vi "Dashboard Main.vi"() -> ()   [LabVIEW 2014]
uses:
  <vilib>/event_ctls.llb/eventvkey.ctl
  <vilib>/Rock Robotics/WPI/Dashboard/WPI_DashboardLogging Global.vi
  <vilib>/Rock Robotics/Network Tables/SD Write Numeric Array.vi
  <vilib>/Rock Robotics/Network Tables/SD Read Number.vi
  <vilib>/Rock Robotics/Network Tables/SD Write Number.vi
  <vilib>/Utility/config.llb/Write Key (String).vi
  <vilib>/Utility/config.llb/Write Key (I32).vi
  <vilib>/Utility/config.llb/NI_LVConfig.lvlib
panel:
  out "RobotIP":string
  in  "TCP":refnum<k5>
  in  "Rec Mode":enum32{"Stop", "Record", "Playback"}(radio)
  in  "Vision":u16(ring)=3 items=["Camera Off", "USB Camera SW", "USB Camera HW", "IP Camera"]
  out "Camera IP":string
  out "Image Message":string="Timeout in Camera Communications"
  in  "Dashboard Tab":T1(tab)
  in  "Switch cameras":bool
  in  "Ring Light Color":T2={"Hue"={42.0, 143.0}, "Sat"={103.21428571428572, 255.0}, "Val"={103.0, 255.0}} {"Hue" scale=0.0..255.0 scale format="%#_3g"}
  in  "Switch to Binary":bool
  in  "Camera Settings":T3={"Frame Rate"=30, "Compression"=30, "Size"=1} {"Frame Rate" scale=1.0..30.0; "Size" items=["640x480", "320x240", "160x120"]}
  out "MotorChart R":cluster{"Numeric":dbl, "Numeric":dbl}(graph)
  out "MotorChart L":T4(graph)
  out "MotorSliders R":cluster{"MotorSlide1":dbl, "MotorSlide2":dbl} {"MotorSlide2" scale=-1.0..1.0 scale format="%#_2e"; "MotorSlide1" scale=-1.0..1.0 scale format="%#_2e"}
  out "MotorSliders L":T5 {"MotorSlide4 2" scale=0.0..14.0 scale format="%#_2e"; "MotorSlide2" scale=-1.0..1.0 scale format="%#_2e"; "MotorSlide1" scale=-1.0..1.0 scale format="%#_2e"}
  out "JS1 Z":dbl(slide) scale=-1.0..1.0 scale format="%#_2e"
  out "JS1 Graph":cluster{"X":dbl, "Y":dbl}[](graph)
  out "JS1 Buttons":T6
  out "JS2 Z":dbl(slide) scale=-1.0..1.0 scale format="%#_2e"
  out "JS2 Graph":cluster{"X":dbl, "Y":dbl}[](graph)
  out "JS2 Buttons":T6
  out "Mode":T7(ring)=enum."Auto Disabled"
  in  "DB Camera Config":bool
  out "fps":dbl format="%#.1g"
  out "Mbps":dbl format="%#.1g"
  out "Mbps 2":bool
  in  "DB/String 9":string
  in  "DB/String 8":string
  in  "DB/String 7":string
  in  "DB/String 6":string
  in  "DB/String 5":string
  in  "DB/String 4":string
  in  "DB/String 3":string
  in  "DB/String 2":string
  in  "DB/String 1":string
  in  "DB/String 0":string
  in  "DB/Slider 0":dbl(slide) scale=0.0..5.0
  in  "DB/Slider 1":dbl(slide) scale=0.0..5.0
  in  "DB/Slider 2":dbl(slide) scale=0.0..5.0
  in  "DB/Slider 3":dbl(slide) scale=0.0..5.0
  out "DB/LED 3":bool
  out "DB/LED 2":bool
  out "DB/LED 1":bool
  out "DB/LED 0":bool
  in  "DB/Button 3":bool
  in  "DB/Button 2":bool
  in  "DB/Button 1":bool
  in  "DB/Button 0":bool caption="New Name"
  out "gyro":dbl
  in  "# totes":dbl=1.0
  out "ultrasonic":dbl
  out "pot value":dbl
  in  "lift pid gains":dbl[](array[numeric])=[5.0, 0.0, 0.0]
  in  "Min lift output":dbl=0.2
  out "VROOM METER":dbl(knob) scale=0.0..10.0
  in  "Level setpoints":dbl[](array[numeric])=[0.6, 0.64, 0.79, 0.85]
  in  "lift lower limit":dbl=0.59
  in  "lift upper limit":dbl=0.86
  in  "proportional constant":dbl=11.0
  in  "Test Slider":dbl(slide) scale=0.0..100.0 scale format="%#_3g"
  in  "On/Off":bool caption="Solenoid"
  in  "Test Name":u16(ring) items=["Select the test to run...", "Example Test", "-------------------------------", "List of tests is built in robot code.", "Replace with your own automated tests."]
  in  "Test Tree":string(tree)
  in  "Motor":cluster{"Value":dbl, "Enable":bool} {"Value" scale=-1.0..1.0 scale format="%#_3g"}
  out "Progress":T8 {"Test Progress" scale=0.0..100.0}
  in  "Rev/Fwd":cluster{"Forward":bool, "Reverse":bool}
  in  "Test Ring":u16(ring) items=["Monochrome", "Color"]
  in  "Listbox":i32(listbox)
  out "Tree":string(tree)
  out "Camera Image":T9(plugin-control)
  out "Boolean":bool
  # "Left"
  # "Front"
  # "Right"
  # "Battery"
  # ":l"
  # ":)"
  # ":D"
  # ":/"
  # "VROOM!!!!!!"
  # ":("
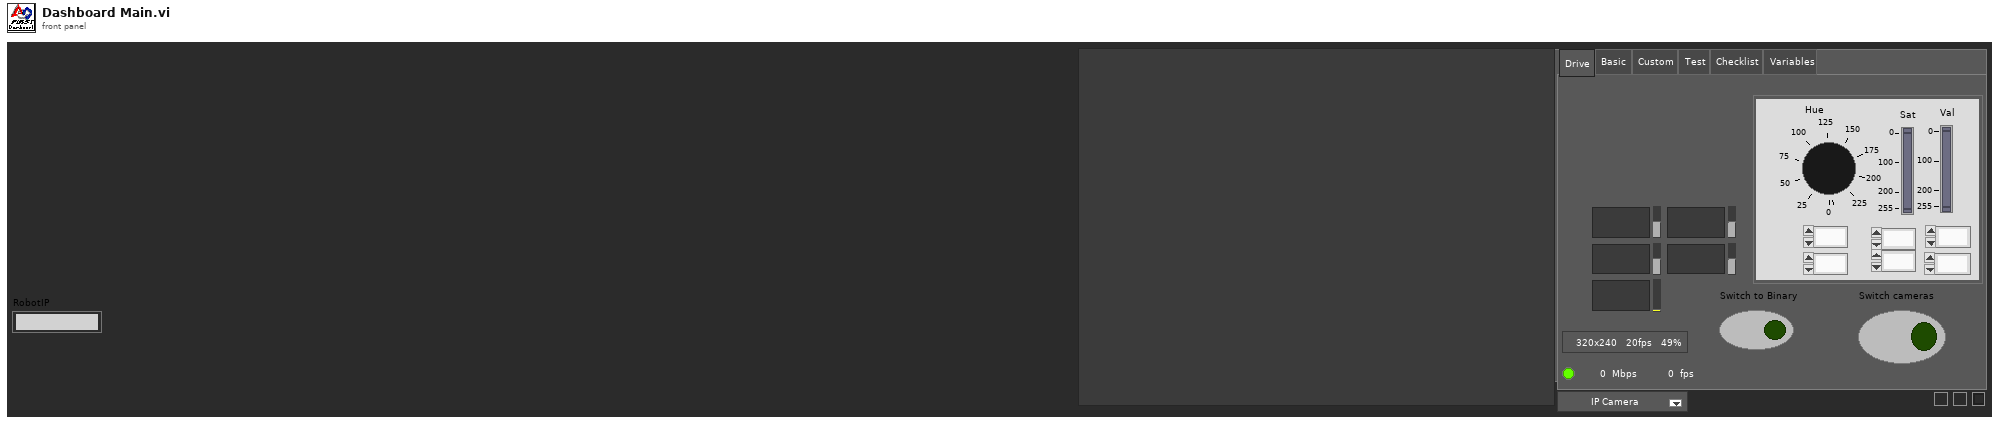
[diagram p1: front panel]
types:
  T1 = enum32{"Drive", "Basic", "Custom", "Test", "Checklist", "Variables"}
  T2 = cluster{"Hue":cluster{dbl, dbl}, "Sat":cluster{dbl, dbl}, "Val":cluster{dbl, dbl}}
  T3 = cluster{"Frame Rate":i32, "Compression":i32, "Size":u16}
  T4 = cluster{"Numeric":dbl, "Numeric":dbl, "Battery V":dbl}
  T5 = cluster{"MotorSlide1":dbl, "MotorSlide2":dbl, "MotorSlide4 2":dbl}
  T6 = cluster{bool, bool, bool, bool, bool, bool, bool, bool, bool, bool, bool, bool}
  T7 = enum8{"Tele-Op Disabled", "Tele-Op Enabled", "Auto Disabled", "Auto Enabled", "Test Disabled", "Test Enabled", "Disconnected", "No Code", "E-Stop"}
  T8 = cluster{"Test Progress":u8, "Test Progress Text":string}
  T9 = typedef "IMAQ Image.ctl" = refnum<image>
  T10 = typedef "Image Type" = u32
  T11 = cluster{"Camera Image":refnum<vi>, "Dashboard Tab":refnum<vi>, "Boolean":refnum<vi>, "Vision":refnum<vi>, "Rec Mode":refnum<vi>, "Test Slider":refnum<vi>, "On/Off ":refnum<vi>, "Test Ring":refnum<vi>, "Rev/Fwd":refnum<vi>, "Test Name":refnum<vi>, "Motor":refnum<vi>, "Progress":refnum<vi>, "CheckList":refnum<vi>, "Tree":refnum<vi>, "Test Tree":refnum<vi>}
  T12 = cluster{"Total Center of Mass":cluster{"X":dbl, "Y":dbl}, "average distance":dbl}
  T13 = cluster{"Error Strings":string, "Disable Counts":cluster{u16, u16}, "Rail Faults":cluster{u16, u16, u16}, "Robot IP":string, "DB Mode":u8, "Event Info":cluster{"Name":string, "Type":u8, "Number":u16, "Replay":u8}, "Camera Addr":string}
  T14 = cluster{"Storage":cluster{"Disk Free":u64, "RAM Block":u32, "RAM free":u32}, "CPU Utilization":cluster{"CPU % ISR":sgl, "CPU % Time Crit":sgl, "CPU % Timed Str":sgl, "CPU % High":sgl, "CPU % Above":sgl, "CPU % Normal":sgl, "CPU % Low":sgl}, "CAN":cluster{"% Bus Utilization":sgl, "Bus Off Cnt":u32, "TX_FIFO Full Cnt":u32, "Receive Error Cnt":u8, "Transmit Error Cnt":u8}, "HID":cluster{"HID Outputs":u32, "Rumble Low":u16, "Rumble High":u16}[]}
  T15 = cluster{"Status bits":cluster{"Test Mode":bool, "Autonomous":bool, "Enabled":bool, "Code Start":bool, "Brownout":bool, "Reserved 2":bool, "Reserved 3":bool, "E-Stop":bool}, "Code Trace":cluster{"Disabled":bool, "TeleOp":bool, "Auto":bool, "Test":bool}, "Controller Type":enum16{"unknown", "cRIO", "roboRio"}, "Code?":enum16{"unknown", "noCode", "code"}, "Battery V":dbl}
  T16 = cluster{"Control Bits":cluster{"TestMode":bool, "Autonomous":bool, "Enabled":bool, "FMS Present":bool, bool, bool, bool, "E-Stop":bool}, "Team Station ":u8, "Countdown":sgl, "Joystick Values":cluster{"Axes":dbl[], "Buttons":bool[], "POVs":i16[]}[]}
  T17 = cluster{"Axes":dbl[], "Buttons":bool[], "POVs":i16[]}[]
  T18 = cluster{"Axes":dbl[], "Buttons":bool[], "POVs":i16[]}
  T19 = cluster{"Buttons[0]":bool, "Buttons[1]":bool, "Buttons[2]":bool, "Buttons[3]":bool, "Buttons[4]":bool, "Buttons[5]":bool, "Buttons[6]":bool, "Buttons[7]":bool, "Buttons[8]":bool, "Buttons[9]":bool, "Buttons[10]":bool, "Buttons[11]":bool}
  T20 = typedef "NI_LVConfig.lvlib/Config Data RefNum.ctl" = refnum<k1>
  T21 = cluster{"Operation":enum16{"Update", "Clear"}, "Color Box":u32}[]
  T22 = typedef "eventvkey.ctl" = enum16{"ASCII", "Enter", "Return", "Shift", "Ctrl", "Alt", "Cmd", "Opt", "Caps", "NumLock", "Clear", "Break", "Up", "Down", "Left", "Right", "Insert", "Delete", "Home", "End", "PageUp", "PageDown", "Escape", "Help", "Pause", "ScrollLock", "F1", "F2", "F3", "F4", "F5", "F6", "F7", "F8", "F9", "F10", "F11", "F12", "F13", "F14", "F15", "F16", "F17", "F18", "F19", "F20", "F21", "F22", "F23", "F24", "Play", "VolumeUp", "VolumeDown", "Mute", "Two Byte Char"}
  T23 = cluster{"Image Size":bool, "Image Type":bool, "Pixel Value":bool, "ROI Information":bool, "Zoom Factor":bool}
  T24 = enum8{"Enabled", "Disabled", "Disabled and Grayed Out"}
  T25 = cluster{"Operation":enum16{"Update", "Clear"}, "Color Box":u32}
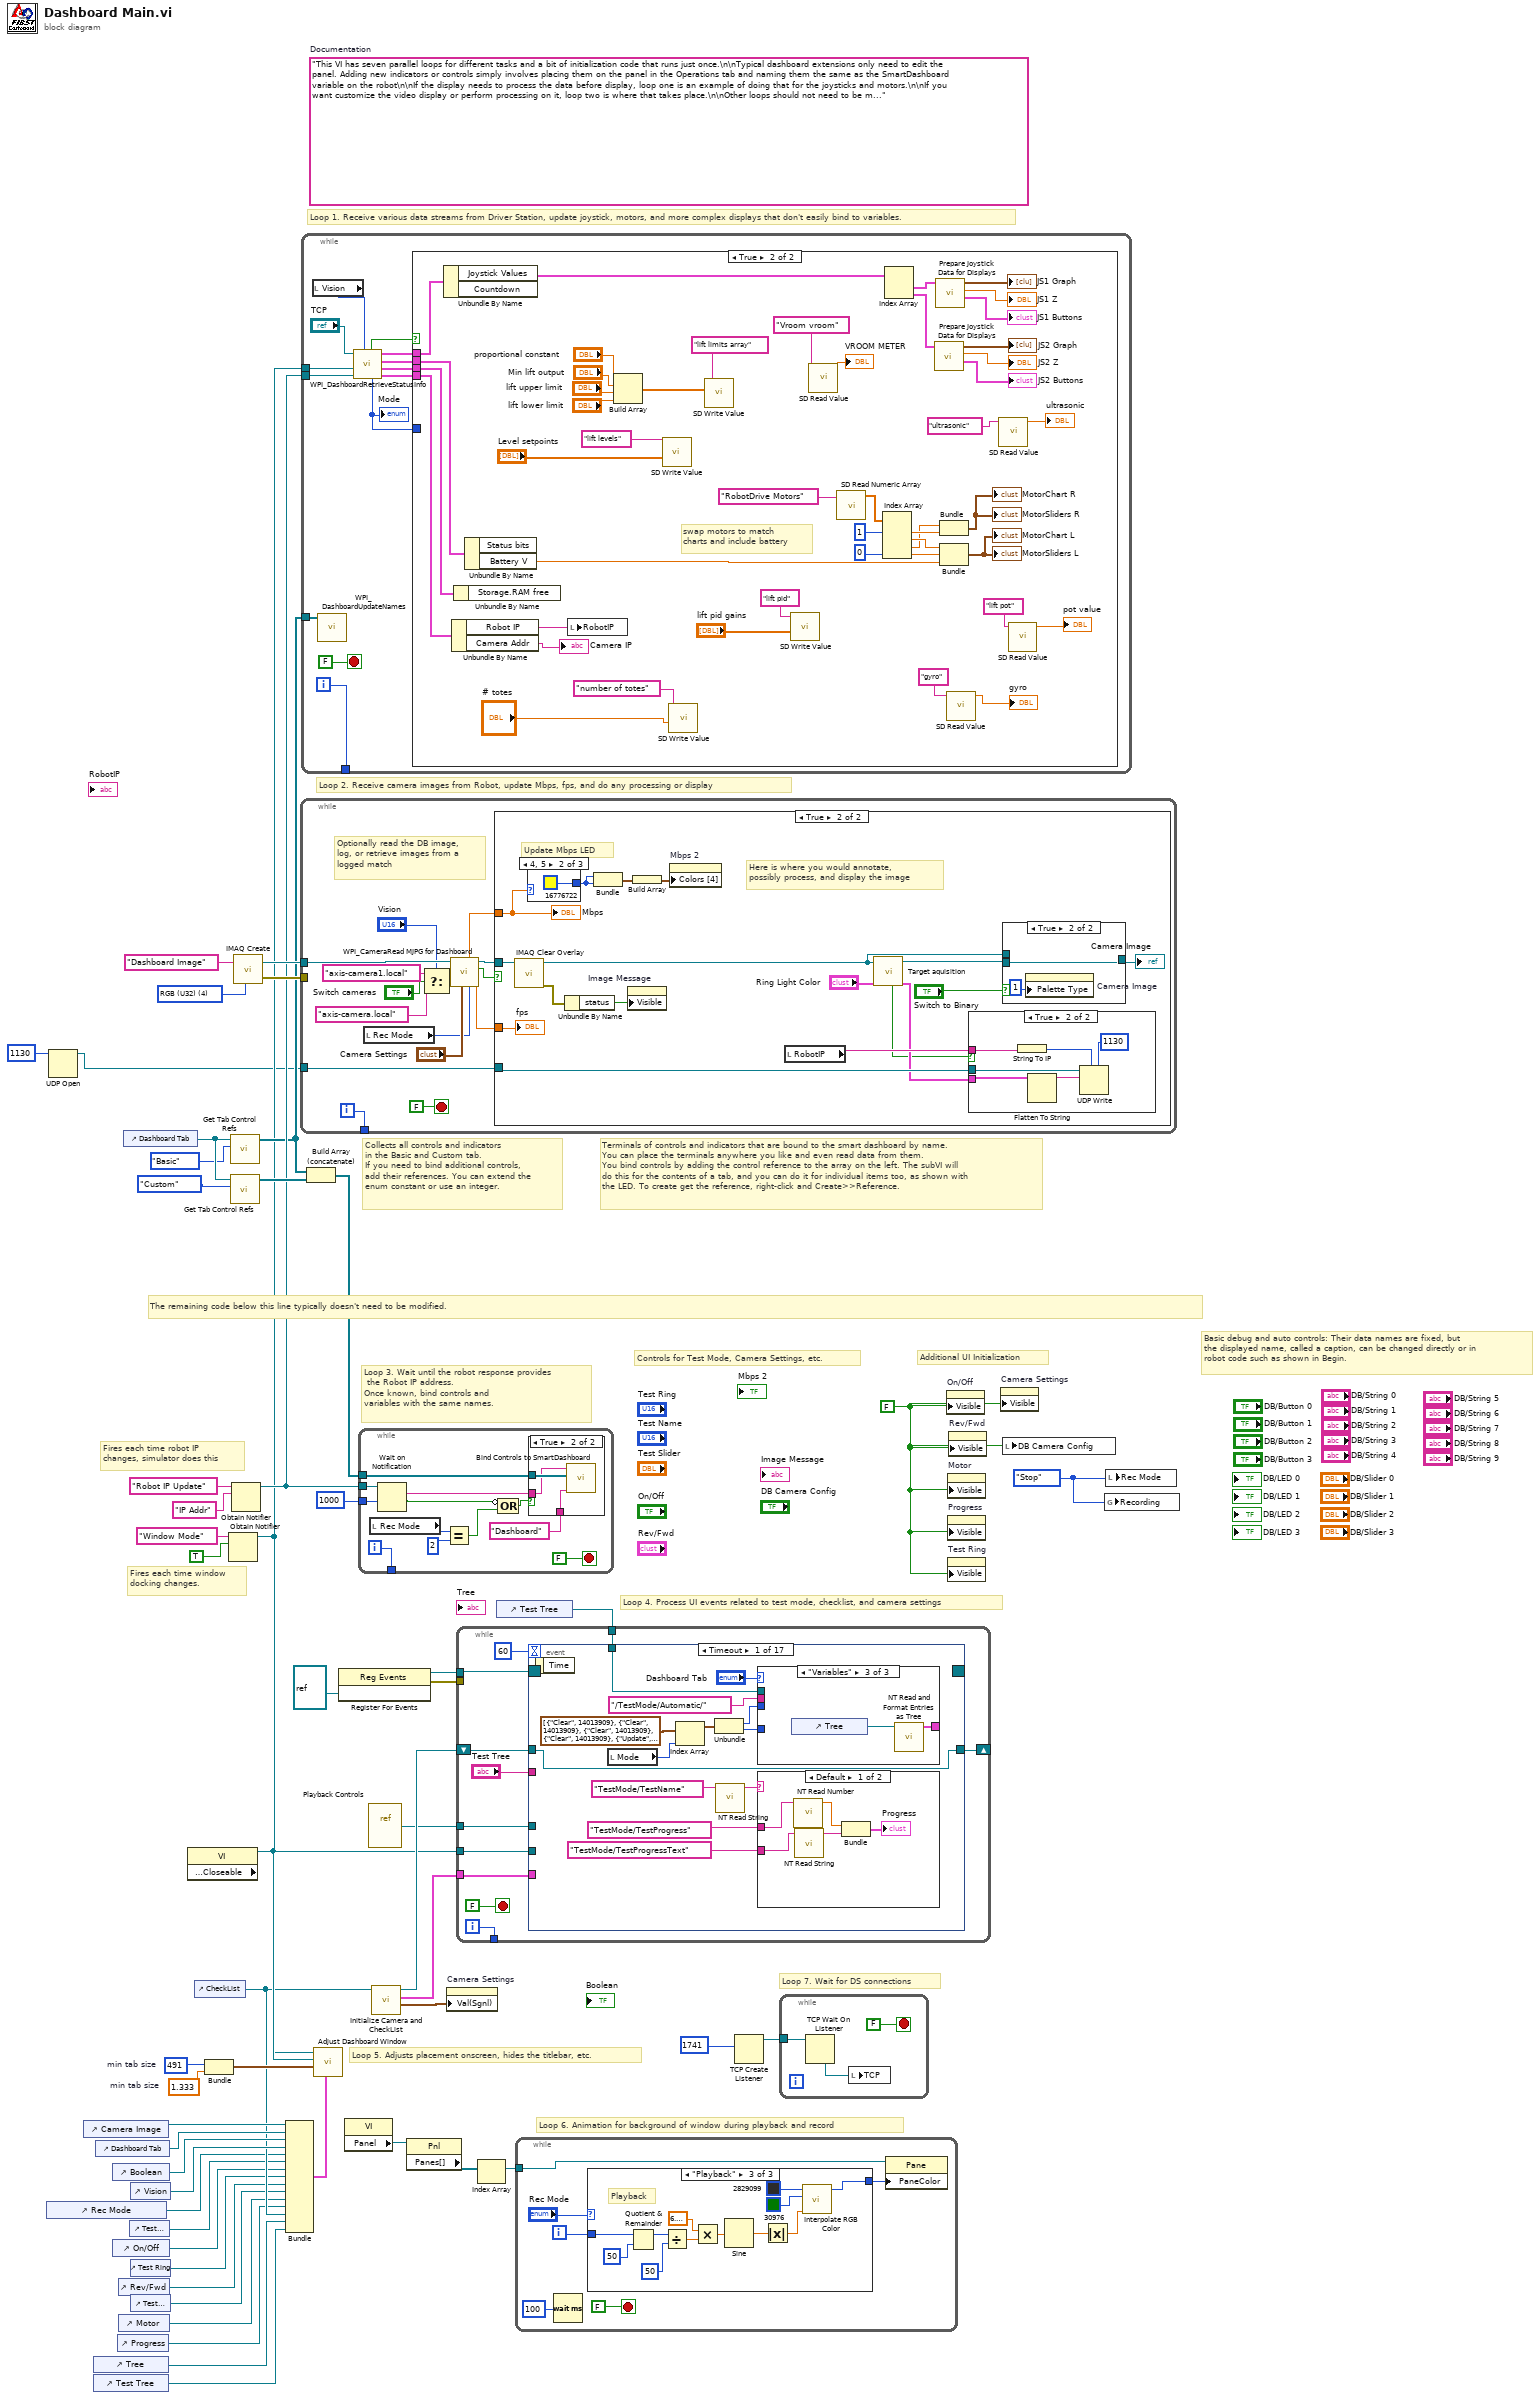
[diagram p0: block diagram]
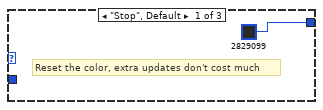
[diagram p3: hidden frame]
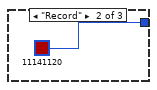
[diagram p4: hidden frame]
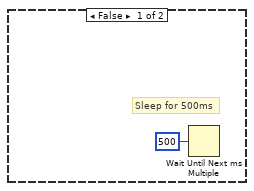
[diagram p6: hidden frame]
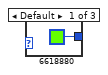
[diagram p9: hidden frame]
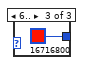
[diagram p10: hidden frame]
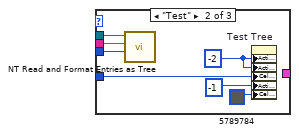
[diagram p12: hidden frame]
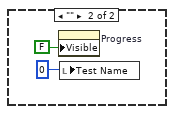
[diagram p13: hidden frame]
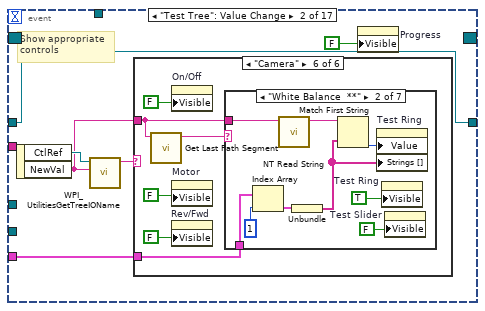
[diagram p14: hidden frame]
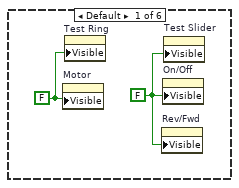
[diagram p15: hidden frame]
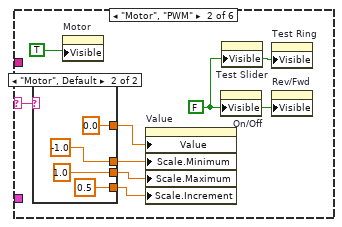
[diagram p16: hidden frame]
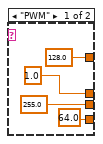
[diagram p17: hidden frame]
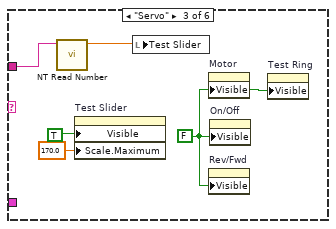
[diagram p18: hidden frame]
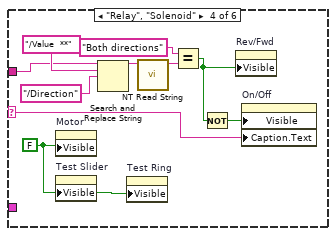
[diagram p19: hidden frame]
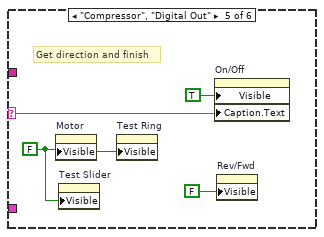
[diagram p20: hidden frame]
diagram:
  w26 = 491  # min tab size
  w25 = 1.333  # min tab size
  w34 = enum32{"Stop", "Record", "Playback"}."Stop" ("Rec Mode")
  w8 = FALSE ("Visible")
  (unwired) "This VI has seven parallel loops for different tasks and a bit of initialization code that runs just once.\n\nTypical dashboard extensions only need to edit the panel. Adding new indicators or controls simply involves placing them on the panel in the Operations tab and naming them the same as the SmartDashboard variable on the robot\n\nIf the display needs to process the data before display, loop one is an example of doing that for the joysticks and motors.\n\nIf you want customize the video display or perform processing on it, loop two is where that takes place.\n\nOther loops should not need to be modified. They are pretty standard, and document the task they perform."  # Documentation
  w54 = T10 4 items=["Grayscale (U8)", "Grayscale (I16)", "Grayscale (SGL)", "Complex (CSG)", "RGB (U32)", "HSL (U32)", "RGB (U64)"] ("Image Type")
  # "Loop 7. Wait for DS connections"
  # "Basic debug and auto controls: Their data names are fixed, but\nthe displayed name, called a caption, can be changed directly or in\nrobot code such as shown in Begin."
  # "Controls for Test Mode, Camera Settings, etc."
  # "Additional UI Initialization"
  # "Loop 6. Animation for background of window during playback and record"
  # "Fires each time robot IP\nchanges, simulator does this"
  # "Fires each time window\ndocking changes."
  # "Collects all controls and indicators\nin the Basic and Custom tab.\nIf you need to bind additional controls,\nadd their references. You can extend the\nenum constant or use an integer."
  # "The remaining code below this line typically doesn't need to be modified."
  # "Loop 4. Process UI events related to test mode, checklist, and camera settings"
  # "Terminals of controls and indicators that are bound to the smart dashboard by name.\nYou can place the terminals anywhere you like and even read data from them.\nYou bind controls by adding the control reference to the array on the left. The subVI will\ndo this for the contents of a tab, and you can do it for individual items too, as shown with\nthe LED. To create get the reference, right-click and Create>>Reference."
  # "Loop 3. Wait until the robot response provides\n the Robot IP address.\nOnce known, bind controls and\nvariables with the same names."
  # "Loop 5. Adjusts placement onscreen, hides the titlebar, etc."
  # "Loop 1. Receive various data streams from Driver Station, update joystick, motors, and more complex displays that don't easily bind to variables."
  # "Loop 2. Receive camera images from Robot, update Mbps, fps, and do any processing or display"
  n1 = control-ref of="Rec Mode"() -> (w14:refnum<vi>)
  n2 = UDP Open(11:1130) -> (port=w1:refnum<k16>)  [unwired: 4 in, 2 out]
  n3 = control-ref of="Camera Image"() -> (w29:refnum<vi>)
  n4 = control-ref of="Tree"() -> (w18:refnum<vi>)
  n5 = control-ref of="Test Tree"() -> (w17:refnum<vi>)
  n6 = control-ref of="Dashboard Tab"() -> (w28:refnum<vi>)
  n7 = control-ref of="Boolean"() -> (w23:refnum<vi>)
  n8 = control-ref of="On/Off"() -> (w12:refnum<vi>)
  n9 = control-ref of="Progress"() -> (w9:refnum<vi>)
  n10 = control-ref of="Rev/Fwd"() -> (w10:refnum<vi>)
  n11 = control-ref of="Motor"() -> (w15:refnum<vi>)
  n12 = control-ref of="Dashboard Tab"() -> (w32:refnum<vi>)
  n13 = control-ref of="Test Slider"() -> (w13:refnum<vi>)
  n14 = control-ref of="Vision"() -> (w27:refnum<vi>)
  n15 = control-ref of="Test Ring"() -> (w11:refnum<vi>)
  n16 = control-ref of="Test Name"() -> (w16:refnum<vi>)
  n17 = property class="VI" props=["Front Panel.Closeable"]() -> (reference out=w33:refnum<vi>)  [unwired: 2 in, 2 out]
  n18 = control-ref of="CheckList"() -> (w19:refnum<vi>)
  n19 = Bundle("min tab size"=w26, "min tab size"=w25) -> (w24:cluster{"min tab size":i32, "min tab size":dbl})  [unwired: 1 in]
  n20 = Obtain Notifier(name (unnamed)="Window Mode", notification data type=TRUE) -> (notifier out=w5:refnum<notifier>)  [unwired: 2 in, 2 out]
  n21 = call <vilib>:"Get Tab Control Refs.vi"("Page Index"=T1."Basic" ("Dashboard Tab"), "TabControl in"=w32) -> ("ControlsOnPage"=w6:refnum<vi>[])  [unwired: 9 in]
  n22 = call <vilib>:"Get Tab Control Refs.vi"("Page Index"=T1."Custom" ("Dashboard Tab"), "TabControl in"=w32) -> ("ControlsOnPage"=w31:refnum<vi>[])  [unwired: 9 in]
  n23 = Obtain Notifier(name (unnamed)="Robot IP Update", notification data type="IP Addr" ("name (unnamed)")) -> (notifier out=w7:refnum<notifier>)  [unwired: 2 in, 2 out]
  n24 = call "IMAQ Create"("Image Name"="Dashboard Image", "Image Type"=w54) -> ("New Image"=w52:T9, "error out"=w51:errorcluster)  [unwired: 2 in, 1 out]
  n25 = Bundle("Camera Image"=w29, "Dashboard Tab"=w28, "Boolean"=w23, "Vision"=w27, "Rec Mode"=w14, "Test Slider"=w13, "On/Off"=w12, "Test Ring"=w11, "Rev/Fwd"=w10, "Test Name"=w16, "Motor"=w15, "Progress"=w9, "CheckList"=w19, "Tree"=w18, "Test Tree"=w17) -> (w20:T11)  [unwired: 1 in]
  n26 = while {
    tunnel: w52 -> [w67]
    tunnel: w51 -> [_]
    tunnel: [w68] -> _
    tunnel: w1 -> [w59]
    i -> [w68]
    stop <- FALSE stop-if-true
    # "Optionally read the DB image,\nlog, or retrieve images from a\nlogged match"
    n27 = local read "Rec Mode"() -> (w61:enum32{"Stop", "Record", "Playback"})
    n28 = Select(t="axis-camera1.local", s="Switch cameras", f="axis-camera.local") -> (s? t:f=w58:string)
    n29 = call <vilib>:"WPI_CameraRead MJPG for Dashboard.vi"("Camera Settings"="Camera Settings", "Rec Mode"=w61, "Camera IP"=w58, "Camera Mode"="Vision", "Refnum in"=w67) -> ("Active"=w65:bool, "Refnum out"=w66:T9, "FPS"=w64:dbl, "Bandwidth (Mbps)"=w63:dbl)  [unwired: 3 in]
    n30 = case shown="True" w65 {
      tunnel: w66 -> [_ w82]
      tunnel: w63 -> [_ w81]
      tunnel: w64 -> [_ w80]
      tunnel: w59 -> [_ w73]
      frame False {
        # "Sleep for 500ms"
        n31 = Wait Until Next ms Multiple(millisecond multiple=u32 500) -> ()  [unwired: 1 out]
      }
      frame True {
        # "Here is where you would annotate,\npossibly process, and display the image"
        # "Update Mbps LED"
        n32 = call "IMAQ Clear Overlay"("Image"=w82) -> ("error out"=w86:errorcluster, "Image Out"=w78:T9)  [unwired: 2 in, 7 out]
        n33 = case shown="4, 5" w81 {
          tunnel: [u32 6618880 ("Color Box") u32 16776722 ("Color Box") u32 16716800 ("Color Box")] -> w83
          frame Default {
          }
          frame 4, 5 {
          }
          frame 6.. {
          }
        }
        n34 = Unbundle By Name(w86) -> ("status"=w87:bool)
        n35 = Bundle("Color Box"=w83, "Color Box"=w83) -> (w85:cluster{"Color Box":u32, "Color Box":u32})  [unwired: 1 out]
        n36 = property on="Image Message" class="Str"("Visible"=w87) -> ()  [unwired: 2 in, 2 out]
        n37 = Build Array(w85) -> (w84:cluster{"Color Box":u32, "Color Box":u32}[])
        n38 = property on="Mbps 2" class="Bool (strict)"("Colors [4]"=w84) -> ()  [unwired: 2 in, 2 out]
        n39 = local read "RobotIP"() -> (w74:string)
        n40 = call "Target aquisition.vi"("Ring Light Color"="Ring Light Color", "Image"=w78) -> ("Target tracking data"=w72:T12, "Threshold image"=w76:T9, "is there a target"=w71:bool)  [unwired: 7 in]
        n41 = case shown="True" w71 {
          tunnel: w74 -> [_ w91]
          tunnel: w73 -> [_ w90]
          tunnel: w72 -> [_ w88]
          frame False {
          }
          frame True {
            n42 = String To IP(1:w91) -> (0:w92:u32)
            n43 = Flatten To String(anything=w88) -> (data string=w93:string)  [unwired: 3 in, 2 out]
            n44 = UDP Write(address=w92, port or service name=1130, connection ID=w90, data in=w93) -> ()  [unwired: 2 in, 2 out]
          }
        }
        n45 = case shown="True" "Switch to Binary" {
          tunnel: w78 -> [w94 _]
          tunnel: [w94 w95] -> w77
          tunnel: w76 -> [_ w95]
          frame False {
          }
          frame True {
            n46 = property on="Camera Image" class="ImageControl"("Palette Type"=1) -> ()  [unwired: 2 in, 2 out]
          }
        }
        "Camera Image" <- w77
        "Mbps" <- w81
        "fps" <- w80
      }
    }
  }
  n47 = while {
    tunnel: [w111] -> _
    tunnel: w7 -> [w105]
    tunnel: w6 -> [w104]
    tunnel: w5 -> [w100]
    i -> [w111]
    stop <- FALSE stop-if-true
    n48 = local read "Vision"() -> (w102:u16)
    n49 = call <vilib>:"WPI_DashboardUpdateNames.vi"("Controls on Tab"=w104) -> ()  [unwired: 11 in]
    n50 = call <vilib>:"WPI_DashboardRetrieveStatusInfo.vi"("Vision"=w102, "Binding Refnum"=w105, "Window Mode Notifier"=w100, "TCP Cnx"="TCP") -> ("Power and Errors"=w106:T13, "Robot Metrics"=w109:T14, "Status Info"=w110:T15, "Control Info"=w107:T16, "Robot Mode"=w103:T7, "Process?"=w108:bool)  [unwired: 2 in]
    "Mode" <- w103
    n51 = case shown="True" w108 {
      tunnel: w110 -> [_ w158]
      tunnel: w109 -> [_ w157]
      tunnel: w107 -> [_ w156]
      tunnel: w106 -> [_ w155]
      tunnel: w103 -> [_ _]
      frame False {
      }
      frame True {
        # "swap motors to match\ncharts and include battery"
        n52 = Unbundle By Name(w156) -> ("Joystick Values"=w143:T17)  [unwired: 1 out]
        n53 = Unbundle By Name(w155) -> ("Robot IP"=w117:string, "Camera Addr"=→"Camera IP":string)
        n54 = Unbundle By Name(w157) -> ()  [unwired: 1 out]
        n55 = Unbundle By Name(w158) -> ("Battery V"=w144:dbl)  [unwired: 1 out]
        n56 = local write "RobotIP"(w117) -> ()
        n57 = Build Array("proportional constant", "Min lift output", "lift upper limit", "lift lower limit") -> (w130:dbl[])
        n58 = call-poly <vilib>:"SD Write Value.vi"("Numeric Array"="Level setpoints", "Name"="lift levels") -> ()  [unwired: 8 in, 2 out]
        n59 = call-poly <vilib>:"SD Write Value.vi"("Numeric"="# totes", "Name"="number of totes") -> ()  [unwired: 8 in, 2 out]
        n60 = call-poly <vilib>:"SD Write Value.vi"("Numeric Array"=w130, "Name"="lift limits array") -> ()  [unwired: 8 in, 2 out]
        n61 = call-poly <vilib>:"SD Write Value.vi"("Numeric Array"="lift pid gains", "Name"="lift pid") -> ()  [unwired: 8 in, 2 out]
        n62 = call-poly <vilib>:"SD Read Value.vi"("Name"="Vroom vroom") -> ("Numeric"=→"VROOM METER":dbl)  [unwired: 8 in, 2 out]
        n63 = call <vilib>:"SD Read Numeric Array.vi"("Name"="RobotDrive Motors") -> ("Numeric Array"=w146:dbl[])  [unwired: 8 in, 2 out]
        n64 = Index Array(array=w146, index #1=1, index #4=0) -> (element #1=w150:dbl, element #2=w151:dbl, element #3=w149:dbl, element #4=w154:dbl)  [unwired: 2 in]
        n65 = Index Array(array=w143) -> (element #1=w142:T18, element #2=w137:T18)  [unwired: 2 in]
        n66 = call "Prepare Joystick Data for Displays.vi"("Joystick Values"=w137) -> ("Buttons"=→"JS2 Buttons":T19, "Z Axis"=→"JS2 Z":dbl, "Cartesian Data"=→"JS2 Graph":cluster{"X axis":dbl, "X axis":dbl}[])  [unwired: 8 in]
        n67 = call "Prepare Joystick Data for Displays.vi"("Joystick Values"=w142) -> ("Buttons"=→"JS1 Buttons":T19, "Z Axis"=→"JS1 Z":dbl, "Cartesian Data"=→"JS1 Graph":cluster{"X axis":dbl, "X axis":dbl}[])  [unwired: 8 in]
        n68 = Bundle("Numeric"=w149, "Numeric"=w150) -> (→"MotorChart R" →"MotorSliders R":cluster{"Numeric":dbl, "Numeric":dbl})  [unwired: 1 in]
        n69 = Bundle("Numeric"=w151, "Numeric"=w154, "Battery V"=w144) -> (→"MotorChart L" →"MotorSliders L":T4)  [unwired: 1 in]
        n70 = call-poly <vilib>:"SD Read Value.vi"("Name"="gyro") -> ("Numeric"=→"gyro":dbl)  [unwired: 8 in, 2 out]
        n71 = call-poly <vilib>:"SD Read Value.vi"("Name"="ultrasonic") -> ("Numeric"=→"ultrasonic":dbl)  [unwired: 8 in, 2 out]
        n72 = call-poly <vilib>:"SD Read Value.vi"("Name"="lift pot") -> ("Numeric"=→"pot value":dbl)  [unwired: 8 in, 2 out]
      }
    }
  }
  n73 = Build Array (concatenate)(w6, w31) -> (w30:refnum<vi>[])
  n74 = call "Adjust Dashboard Window.vi"("Sizing Refnums"=w20, "Size Constraints"=w24, "VI"=w33, "Notifier in"=w5) -> ()  [unwired: 8 in]
  n75 = register-events(refnum<vi> refnum) -> (reference out=w38:refnum<event-registration>, error out=w37:errorcluster)  [unwired: 2 in]
  n76 = property class="VI"() -> ("Panel"=w41:refnum<vi>)  [unwired: 2 in, 2 out]
  n77 = while {
    tunnel: w30 -> [w170]
    tunnel: w7 -> [w168]
    tunnel: [w166] -> _
    tunnel: u32 1000 ("milliseconds to wait") -> [w165]
    i -> [w166]
    stop <- FALSE stop-if-true
    n78 = local read "Rec Mode"() -> (w161:enum32{"Stop", "Record", "Playback"})
    n79 = Wait on Notification(notifier=w168, timeout in ms (-1)=w165) -> (notification=w167:string, timed out?=w163:bool)  [unwired: 2 in, 2 out]
    n80 = Equal?(x=w161, y=u16 2 ("Rec Mode")) -> (x = y?=w162:bool)
    n81 = Compound Arithmetic op=OR(invert w163, w162) -> (w164:bool)
    n82 = case shown="True" w164 {
      tunnel: w170 -> [_ w173]
      tunnel: w167 -> [_ w172]
      tunnel: "Dashboard" -> [_ w171]
      frame False {
      }
      frame True {
        n83 = call <vilib>:"Bind Controls to SmartDashboard.vi"("Client Name"=w171, "Bound Control Refs"=w173, "Server IP Address"=w172) -> ()  [unwired: 9 in]
      }
    }
  }
  n84 = vi-ref "Playback Controls.vi"() -> (w39:refnum<vi>)
  n85 = call "Initialize Camera and CheckList.vi"("ListBox in"=w19) -> ("Cluster"=w45:cluster{"value":i32, "value":i32, "index":i32}, "Array"=w46:cluster{string[]}[], "File Refnum"=w44:T20)  [unwired: 8 in]
  n86 = property class="Pnl"(reference=w41) -> ("Panes[]"=w42:refnum<vi>[])  [unwired: 1 in, 2 out]
  n87 = property on="Camera Settings" class="Clust (strict)"("Val(Sgnl)"=w45) -> ()  [unwired: 2 in, 2 out]
  n88 = Index Array(array=w42) -> (element=w40:refnum<vi>)  [unwired: 1 in]
  n89 = control-ref of="Test Tree"() -> (w43:refnum<vi>)
  n90 = while {
    tunnel: w46 -> [w181]
    shift-right: [w180] -> _
    shift-left: w44 -> [w179]
    tunnel: [w178] -> _
    tunnel: w43 -> [w177]
    tunnel: w39 -> [w176]
    tunnel: w38 -> [w175]
    tunnel: w37 -> [_]
    tunnel: w33 -> [w174]
    i -> [w178]
    stop <- FALSE stop-if-true
    n91 = event shown="[0] Timeout" {
      selector: w175 -> [_ _ _ _ _ _ _ _ _ _ _ _ _ _ _ _ _]
      dyn-events: [_ _ _ _ _ _ _ _ _ _ _ _ _ w419 _ _ _] -> _
      timeout: u32 60 ("milliseconds to wait") -> [_ _ _ _ _ _ _ _ _ _ _ _ _ _ _ _ _]
      tunnel: w177 -> [w193 _ _ _ _ _ _ _ _ _ _ _ _ _ _ _ _]
      tunnel: "Test Tree" -> [_ _ _ _ _ _ _ _ w388 w396 w398 w402 w410 _ _ _ _]
      tunnel: w181 -> [_ w215 _ _ _ _ w352 w382 _ _ _ _ _ _ _ _ _]
      tunnel: [w189 w214 w313 w318 w326 w338 w351 w375 w387 w394 w397 w401 w409 w421 w435 w436 w446] -> w180
      tunnel: w179 -> [w189 w214 w313 w318 w326 w338 w350 w375 w387 w394 w397 w401 w409 w421 w435 w436 w446]
      tunnel: w176 -> [_ _ _ _ _ _ _ _ _ _ _ _ _ w422 _ w439 _]
      tunnel: w174 -> [_ _ _ _ _ _ _ _ _ _ _ _ _ w417 _ _ _]
      event Timeout {
        n92 = event-data() -> ()  [unwired: 1 in, 1 out]
        n93 = local read "Mode"() -> (w192:T7)
        n94 = Index Array(array=T21 [{"Operation"=enum."Clear", "Color Box"=14013909}, {"Operation"=enum."Clear", "Color Box"=14013909}, {"Operation"=enum."Clear", "Color Box"=14013909}, {"Operation"=enum."Clear", "Color Box"=14013909}, {"Operation"=enum."Update", "Color Box"=14013909}, {"Operation"=enum."Update", "Color Box"=16777215}, {"Operation"=enum."Clear", "Color Box"=14013909}, {"Operation"=enum."Clear", "Color Box"=14013909}, {"Operation"=enum."Clear", "Color Box"=14013909}], index=w192) -> (element=w187:T25)
        n95 = Unbundle(w187) -> ("Operation"=w186:enum16{"Update", "Clear"}, "Color Box"=w185:u32)
        n96 = call <vilib>:"NT Read String.vi"("Name"="TestMode/TestName") -> ("String"=w196:string)  [unwired: 9 in, 1 out]
        n97 = case shown="\"Variables\"" "Dashboard Tab" {
          tunnel: w193 -> [_ w204 _]
          tunnel: "/TestMode/Automatic/" ("Name Pattern") -> [_ w203 _]
          tunnel: w186 -> [_ w202 _]
          tunnel: [_ _ w206] -> _
          tunnel: w185 -> [_ w198 _]
          frame "Custom", Default {
          }
          frame "Test" {
            w201 = -2 ("Active Item:Row Number")
            n98 = call <vilib>:"NT Read and Format Entries as Tree.vi"("Operation"=w202, "Name Pattern"=w203, "Tree Refnum"=w204) -> ()  [unwired: 7 in, 2 out]
            n99 = property on="Test Tree" class="Tree (strict)"("Active Item Row Number"=w201, "ActiveColNum"=w201, "CellBG"=w198, "Active Item Row Number"=-1 ("Active Item:Row Number"), "CellBG"=u32 5789784 ("Color Box")) -> ()  [unwired: 2 in, 2 out]
          }
          frame "Variables" {
            n100 = control-ref of="Tree"() -> (w205:refnum<vi>)
            n101 = call <vilib>:"NT Read and Format Entries as Tree.vi"("Tree Refnum"=w205) -> ("Formatted Strings"=w206:cluster{"Name":string, "Value":string}[])  [unwired: 9 in, 1 out]
          }
        }
        n102 = case shown="Default" w196 {
          tunnel: "TestMode/TestProgress" ("Name") -> [w208 _]
          tunnel: "TestMode/TestProgressText" ("Name") -> [w207 _]
          frame Default {
            n103 = call <vilib>:"NT Read Number.vi"("Name"=w208) -> ("Numeric"=w209:dbl)  [unwired: 9 in, 1 out]
            n104 = call <vilib>:"NT Read String.vi"("Name"=w207) -> ("String"=w210:string)  [unwired: 9 in, 1 out]
            n105 = Bundle("Numeric"=w209, "String"=w210) -> (→"Progress":cluster{"Numeric":dbl, "String":string})  [unwired: 1 in]
          }
          frame "" {
            n106 = property on="Progress" class="Clust (strict)"("Visible"=FALSE) -> ()  [unwired: 2 in, 2 out]
            n107 = local write "Test Name"(u16 0) -> ()
          }
        }
      }
      event "Test Tree": Value Change {
        # "Show appropriate\ncontrols"
        n108 = event-data() -> ("CtlRef"=w218:refnum<vi>, "NewVal"=w216:string)  [unwired: 1 in]
        n109 = call <vilib>:"WPI_UtilitiesGetTreeIOName.vi"("NewVal"=w216, "TreeControl in"=w218) -> ("I/O Name"=w219:string)  [unwired: 9 in]
        n110 = case shown="\"Camera\"" w219 {
          selector: w219 -> [_ w226 _ w244 w253 _]
          tunnel: w216 -> [_ _ w241 w243 _ w260]
          tunnel: w215 -> [_ _ _ _ _ w259]
          frame Default {
            w221 = FALSE ("Visible")
            w220 = FALSE ("Visible")
            n111 = property on="Motor" class="Clust (strict)"("Visible"=w220) -> ()  [unwired: 2 in, 2 out]
            n112 = property on="Test Ring" class="Ring (strict)"("Visible"=w220) -> ()  [unwired: 2 in, 2 out]
            n113 = property on="Rev/Fwd" class="Clust (strict)"("Visible"=w221) -> ()  [unwired: 2 in, 2 out]
            n114 = property on="On/Off" class="Bool (strict)"("Visible"=w221) -> ()  [unwired: 2 in, 2 out]
            n115 = property on="Test Slider" class="Slide (strict)"("Visible"=w221) -> ()  [unwired: 2 in, 2 out]
          }
          frame "Motor", "PWM" {
            w227 = FALSE ("Visible")
            n116 = case shown="\"Motor\", Default" w226 {
              tunnel: [1.0 ("Value") -1.0 ("Value")] -> w225
              tunnel: [255.0 ("Value") 1.0 ("Value")] -> w224
              tunnel: [128.0 ("Value") 0.0 ("Value")] -> w223
              tunnel: [64.0 ("Value") 0.5 ("Value")] -> w222
              frame "PWM" {
              }
              frame "Motor", Default {
              }
            }
            n117 = property on="Motor" class="Clust (strict)"("Visible"=TRUE) -> ()  [unwired: 2 in, 2 out]
            n118 = property on="Value" class="Slide (strict)"("Value"=w223, "Scale.Minimum"=w225, "Scale.Maximum"=w224, "Scale.Increment"=w222) -> ()  [unwired: 2 in, 2 out]
            n119 = property on="On/Off" class="Bool (strict)"("Visible"=w227) -> ()  [unwired: 2 in, 2 out]
            n120 = property on="Test Slider" class="Slide (strict)"("Visible"=w227) -> ()  [unwired: 2 in, 2 out]
            n121 = property on="Test Ring" class="Ring (strict)"("Visible"=w227) -> ()  [unwired: 2 in, 2 out]
            n122 = property on="Rev/Fwd" class="Clust (strict)"("Visible"=w227) -> ()  [unwired: 2 in, 2 out]
          }
          frame "Servo" {
            w239 = FALSE ("Visible")
            n123 = call <vilib>:"NT Read Number.vi"("Name"=w241) -> ("Numeric"=w240:dbl)  [unwired: 9 in, 1 out]
            n124 = property on="Test Slider" class="Slide (strict)"("Visible"=TRUE, "Scale.Maximum"=170.0 ("Scale.Range:Maximum")) -> ()  [unwired: 2 in, 2 out]
            n125 = local write "Test Slider"(w240) -> ()
            n126 = property on="Motor" class="Clust (strict)"("Visible"=w239) -> ()  [unwired: 2 in, 2 out]
            n127 = property on="Rev/Fwd" class="Clust (strict)"("Visible"=w239) -> ()  [unwired: 2 in, 2 out]
            n128 = property on="On/Off" class="Bool (strict)"("Visible"=w239) -> ()  [unwired: 2 in, 2 out]
            n129 = property on="Test Ring" class="Ring (strict)"("Visible"=w239) -> ()  [unwired: 2 in, 2 out]
          }
          frame "Relay", "Solenoid" {
            w242 = FALSE ("Visible")
            n130 = property on="Motor" class="Clust (strict)"("Visible"=w242) -> ()  [unwired: 2 in, 2 out]
            n131 = property on="Test Slider" class="Slide (strict)"("Visible"=w242) -> ()  [unwired: 2 in, 2 out]
            n132 = Search and Replace String(input string=w243, search string="/Value  **", replace string="/Direction") -> (result string=w249:string)  [unwired: 5 in, 3 out]
            n133 = property on="Test Ring" class="Ring (strict)"("Visible"=w242) -> ()  [unwired: 2 in, 2 out]
            n134 = call <vilib>:"NT Read String.vi"("Name"=w249) -> ("String"=w247:string)  [unwired: 9 in, 1 out]
            n135 = Equal?(x="Both directions", y=w247) -> (x = y?=w245:bool)
            n136 = Not(x=w245) -> (.not. x?=w246:bool)
            n137 = property on="Rev/Fwd" class="Clust (strict)"("Visible"=w245) -> ()  [unwired: 2 in, 2 out]
            n138 = property on="On/Off" class="Bool (strict)"("Visible"=w246, "Caption.Text"=w244) -> ()  [unwired: 2 in, 2 out]
          }
          frame "Compressor", "Digital Out" {
            w252 = FALSE ("Visible")
            # "Get direction and finish"
            n139 = property on="Motor" class="Clust (strict)"("Visible"=w252) -> ()  [unwired: 2 in, 2 out]
            n140 = property on="Test Slider" class="Slide (strict)"("Visible"=w252) -> ()  [unwired: 2 in, 2 out]
            n141 = property on="Test Ring" class="Ring (strict)"("Visible"=w252) -> ()  [unwired: 2 in, 2 out]
            n142 = property on="On/Off" class="Bool (strict)"("Visible"=TRUE, "Caption.Text"=w253) -> ()  [unwired: 2 in, 2 out]
            n143 = property on="Rev/Fwd" class="Clust (strict)"("Visible"=FALSE) -> ()  [unwired: 2 in, 2 out]
          }
          frame "Camera" {
            n144 = call <vilib>:"Get Last Path Segment.vi"("String in"=w260) -> ("String out"=w261:string)  [unwired: 10 in]
            n145 = property on="On/Off" class="Bool (strict)"("Visible"=FALSE) -> ()  [unwired: 2 in, 2 out]
            n146 = property on="Motor" class="Clust (strict)"("Visible"=FALSE) -> ()  [unwired: 2 in, 2 out]
            n147 = property on="Rev/Fwd" class="Clust (strict)"("Visible"=FALSE) -> ()  [unwired: 2 in, 2 out]
            n148 = case shown="\"White Balance  **\"" w261 {
              tunnel: w260 -> [w267 w276 w285 w294 w303 _ w309]
              tunnel: w259 -> [w265 w273 w282 w291 w300 _ _]
              frame "Size  **" {
                n149 = Index Array(array=w265) -> (element=w264:cluster{string[]})  [unwired: 1 in]
                n150 = call <vilib>:"NT Read String.vi"("Name"=w267) -> ("String"=w266:string)  [unwired: 9 in, 1 out]
                n151 = Unbundle(w264) -> (w262:string[])
                n152 = Match First String(2:w262, 3:w266) -> (0:w263:i32)  [unwired: 1 out]
                n153 = property on="Test Ring" class="Ring (strict)"("Value"=w263, "Strings []"=w262) -> ()  [unwired: 2 in, 2 out]
                n154 = property on="Test Ring" class="Ring (strict)"("Visible"=TRUE) -> ()  [unwired: 2 in, 2 out]
                n155 = property on="Test Slider" class="Slide (strict)"("Visible"=FALSE) -> ()  [unwired: 2 in, 2 out]
              }
              frame "White Balance  **" {
                n156 = Index Array(array=w273, index=1) -> (element=w274:cluster{string[]})
                n157 = call <vilib>:"NT Read String.vi"("Name"=w276) -> ("String"=w275:string)  [unwired: 9 in, 1 out]
                n158 = Unbundle(w274) -> (w271:string[])
                n159 = Match First String(2:w271, 3:w275) -> (0:w270:i32)  [unwired: 1 out]
                n160 = property on="Test Ring" class="Ring (strict)"("Value"=w270, "Strings []"=w271) -> ()  [unwired: 2 in, 2 out]
                n161 = property on="Test Ring" class="Ring (strict)"("Visible"=TRUE) -> ()  [unwired: 2 in, 2 out]
                n162 = property on="Test Slider" class="Slide (strict)"("Visible"=FALSE) -> ()  [unwired: 2 in, 2 out]
              }
              frame "Exposure  **" {
                n163 = Index Array(array=w282, index=2) -> (element=w283:cluster{string[]})
                n164 = call <vilib>:"NT Read String.vi"("Name"=w285) -> ("String"=w284:string)  [unwired: 9 in, 1 out]
                n165 = Unbundle(w283) -> (w279:string[])
                n166 = Match First String(2:w279, 3:w284) -> (0:w280:i32)  [unwired: 1 out]
                n167 = property on="Test Ring" class="Ring (strict)"("Value"=w280, "Strings []"=w279) -> ()  [unwired: 2 in, 2 out]
                n168 = property on="Test Ring" class="Ring (strict)"("Visible"=TRUE) -> ()  [unwired: 2 in, 2 out]
                n169 = property on="Test Slider" class="Slide (strict)"("Visible"=FALSE) -> ()  [unwired: 2 in, 2 out]
              }
              frame "Exposure Priority  **" {
                n170 = Index Array(array=w291, index=3) -> (element=w292:cluster{string[]})
                n171 = call <vilib>:"NT Read String.vi"("Name"=w294) -> ("String"=w293:string)  [unwired: 9 in, 1 out]
                n172 = Unbundle(w292) -> (w288:string[])
                n173 = Match First String(2:w288, 3:w293) -> (0:w289:i32)  [unwired: 1 out]
                n174 = property on="Test Ring" class="Ring (strict)"("Value"=w289, "Strings []"=w288) -> ()  [unwired: 2 in, 2 out]
                n175 = property on="Test Ring" class="Ring (strict)"("Visible"=TRUE) -> ()  [unwired: 2 in, 2 out]
                n176 = property on="Test Slider" class="Slide (strict)"("Visible"=FALSE) -> ()  [unwired: 2 in, 2 out]
              }
              frame "Color Enable  **" {
                n177 = Index Array(array=w300, index=4) -> (element=w301:cluster{string[]})
                n178 = call <vilib>:"NT Read String.vi"("Name"=w303) -> ("String"=w302:string)  [unwired: 9 in, 1 out]
                n179 = Unbundle(w301) -> (w297:string[])
                n180 = Match First String(2:w297, 3:w302) -> (0:w298:i32)  [unwired: 1 out]
                n181 = property on="Test Ring" class="Ring (strict)"("Value"=w298, "Strings []"=w297) -> ()  [unwired: 2 in, 2 out]
                n182 = property on="Test Ring" class="Ring (strict)"("Visible"=TRUE) -> ()  [unwired: 2 in, 2 out]
                n183 = property on="Test Slider" class="Slide (strict)"("Visible"=FALSE) -> ()  [unwired: 2 in, 2 out]
              }
              frame Default {
                n184 = property on="Test Ring" class="Ring (strict)"("Visible"=FALSE) -> ()  [unwired: 2 in, 2 out]
                n185 = property on="Test Slider" class="Slide (strict)"("Visible"=FALSE) -> ()  [unwired: 2 in, 2 out]
              }
              frame "Brightness  **", "Color Level  **", "Compression  **", "FPS  **", "Sharpness  **" {
                n186 = call <vilib>:"NT Read Number.vi"("Name"=w309) -> ("Numeric"=w308:dbl)  [unwired: 9 in, 1 out]
                n187 = local write "Test Slider"(w308) -> ()
                n188 = property on="Test Slider" class="Slide (strict)"("Visible"=TRUE, "Scale.Maximum"=100.0 ("Scale.Range:Maximum")) -> ()  [unwired: 2 in, 2 out]
                n189 = property on="Test Ring" class="Ring (strict)"("Visible"=FALSE) -> ()  [unwired: 2 in, 2 out]
              }
            }
          }
        }
        n190 = property on="Progress" class="Clust (strict)"("Visible"=FALSE) -> ()  [unwired: 2 in, 2 out]
      }
      event "Test Name": Mouse Enter {
        # "Populate the ring with the list of tests"
        n191 = event-data() -> ()  [unwired: 1 in, 1 out]
        n192 = call <vilib>:"NT Read String Array.vi"("Name"="TestMode/TestList") -> ("String Array"=w317:string[])  [unwired: 9 in, 1 out]
        n193 = Build Array (concatenate)("Select the test to run...", w317) -> (w316:string[])
        n194 = property on="Test Name" class="Ring (strict)"("Strings []"=w316) -> ()  [unwired: 2 in, 2 out]
      }
      event "Test Name": Value Change {
        w319 = FALSE ("Visible")
        # "Tell the robot the test name to run"
        n195 = event-data() -> ("NewVal"=w323:u16)  [unwired: 1 in]
        n196 = property on="Test Name" class="Ring (strict)"() -> ("Strings []"=w324:string[])  [unwired: 2 in, 2 out]
        n197 = local write "Progress"(T8 {"Test Progress"=0, "Test Progress Text"=""} ("Progress")) -> ()
        n198 = Index Array(array=w324, index=w323) -> (element=w322:string)
        n199 = call <vilib>:"NT Write String.vi"("String"=w322, "Name"="TestMode/TestName") -> ()  [unwired: 9 in, 1 out]
        n200 = property on="Progress" class="Clust (strict)"("Visible"=TRUE) -> ()  [unwired: 2 in, 2 out]
        n201 = property on="Motor" class="Clust (strict)"("Visible"=w319) -> ()  [unwired: 2 in, 2 out]
        n202 = property on="Test Slider" class="Slide (strict)"("Visible"=w319) -> ()  [unwired: 2 in, 2 out]
        n203 = property on="On/Off" class="Bool (strict)"("Visible"=w319) -> ()  [unwired: 2 in, 2 out]
        n204 = property on="Rev/Fwd" class="Clust (strict)"("Visible"=w319) -> ()  [unwired: 2 in, 2 out]
        n205 = property on="Test Ring" class="Ring (strict)"("Visible"=w319) -> ()  [unwired: 2 in, 2 out]
      }
      event "Listbox": Double Click {
        # "Shift clears all"
        # "Update symbols on the listbox"
        n206 = event-data() -> ("PlatMods.Shift"=w327:bool, "Row"=w329:i32)  [unwired: 1 in]
        n207 = case shown="True" w327 {
          tunnel: w329 -> [w333 _]
          tunnel: 1 -> [w332 _]
          frame False {
            n208 = property on="Listbox" class="LstBox (strict)"() -> ("Item Symbols"=w331:i32[])  [unwired: 2 in, 2 out]
            n209 = Replace Array Subset(array=w331, new element=w332, index=w333) -> (w330:i32[])
            n210 = property on="Listbox" class="LstBox (strict)"("Item Symbols"=w330) -> ()  [unwired: 2 in, 2 out]
          }
          frame True {
            w334 = 0 ("Top Row")
            n211 = property on="Listbox" class="LstBox (strict)"() -> ("Number of Rows"=w336:u32)  [unwired: 2 in, 2 out]
            n212 = Initialize Array(0, w336) -> (w335:i32[])
            n213 = property on="Listbox" class="LstBox (strict)"("Top Row"=w334, "Value"=w334, "Item Symbols"=w335) -> ()  [unwired: 2 in, 2 out]
          }
        }
      }
      event "Listbox": Key Down {
        # "Update symbols on the listbox\nLeft and right keys check and uncheck"
        n214 = event-data() -> ("VKey"=w340:T22)  [unwired: 1 in]
        n215 = case shown="\"Left\", \"Right\"" w340 {
          selector: w340 -> [w345 _]
          tunnel: eventvkey."Left" ("VKey") -> [w343 _]
          frame "Left", "Right" {
            n216 = Equal?(x=w343, y=w345) -> (x = y?=w344:bool)
            n217 = Select(t=0, s=w344, f=1) -> (s? t:f=w346:i32)
            n218 = property on="Listbox" class="LstBox (strict)"() -> ("Item Symbols"=w349:i32[])  [unwired: 2 in, 2 out]
            n219 = Replace Array Subset(array=w349, new element=w346, index="Listbox") -> (w348:i32[])
            n220 = property on="Listbox" class="LstBox (strict)"("Item Symbols"=w348) -> ()  [unwired: 2 in, 2 out]
          }
          frame Default {
          }
        }
      }
      event "DB Camera Config": Value Change {
        # "Show or hide the cluster of controls, store in ini file"
        n221 = event-data() -> ("NewVal"=w353:bool)  [unwired: 1 in]
        n222 = case shown="False" w353 {
          tunnel: w352 -> [w362 _]
          tunnel: [w355 w373] -> w351
          tunnel: w350 -> [w354 w373]
          frame False {
            w369 = "Camera"
            w372 = FALSE ("Visible")
            n223 = local read "Camera Settings"() -> (w361:T3)
            n224 = Index Array(array=w362) -> (element=w365:cluster{string[]})  [unwired: 1 in]
            n225 = Unbundle(w361) -> ("Frame Rate"=w360:i32, "Compression"=w359:i32, "Size"=w363:u16)
            n226 = Unbundle(w365) -> (w364:string[])
            n227 = Index Array(array=w364, index=w363) -> (element=w358:string)
            n228 = call-poly <vilib>:"Write Key.vi"("section"=w369, "value"=w358, "key"="Size", "refnum"=w354) -> ("refnum out"=w371:T20)  [unwired: 2 in, 5 out]
            n229 = call-poly <vilib>:"Write Key.vi"("section"=w369, "value"=w360, "key"="FrameRate", "refnum"=w371) -> ("refnum out"=w370:T20)  [unwired: 1 in, 6 out]
            n230 = property on="Camera Settings" class="Clust (strict)"("Visible"=w372) -> ()  [unwired: 2 in, 2 out]
            n231 = local write "DB Camera Config"(w372) -> ()
            n232 = call-poly <vilib>:"Write Key.vi"("section"=w369, "value"=w359, "key"="Compression", "refnum"=w370) -> ("refnum out"=w356:T20)  [unwired: 1 in, 6 out]
            n233 = call <vilib>:"Close Config Data.vi"("refnum"=w356) -> ("file path"=w357:path)  [unwired: 2 in, 8 out]
            n234 = call <vilib>:"Open Config Data.vi"("configuration file path"=w357) -> ("refnum"=w355:T20)  [unwired: 8 in, 2 out]
          }
          frame True {
            n235 = property on="Camera Settings" class="Clust (strict)"("Visible"=TRUE) -> ()  [unwired: 2 in, 2 out]
          }
        }
      }
      event "Camera Settings": Value Change {
        # "Update summary string when any elements of DB camera change"
        n236 = event-data() -> ("NewVal"=w386:T3)  [unwired: 1 in]
        n237 = Index Array(array=w382) -> (element=w381:cluster{string[]})  [unwired: 1 in]
        n238 = Unbundle(w386) -> ("Frame Rate"=w377:i32, "Compression"=w376:i32, "Size"=w379:u16)
        n239 = Unbundle(w381) -> (w380:string[])
        n240 = Index Array(array=w380, index=w379) -> (element=w378:string)
        n241 = Format Into String(format string="%s   %dfps   %d%%", w378, w377, w376) -> (resulting string=w383:string)  [unwired: 2 in, 1 out]
        n242 = Build Array(w383) -> (w384:string[])
        n243 = property on="DB Camera Config" class="Bool (strict)"("Strings [4]"=w384) -> ()  [unwired: 2 in, 2 out]
      }
      event "Motor.Enable": Value Change {
        # "When the test mode otor enable helper is set, update that\ntree row item's value"
        n244 = event-data() -> ("NewVal"=w392:bool)  [unwired: 1 in]
        n245 = Unbundle("Motor") -> ("Value"=w391:dbl)  [unwired: 1 out]
        n246 = Select(t=w391, s=w392, f=0.0) -> (s? t:f=w389:dbl)
        n247 = call <vilib>:"NT Write Number.vi"("Numeric"=w389, "Name"=w388) -> ()  [unwired: 9 in, 1 out]
      }
      event "Test Slider": Value Change {
        # "When the test mode slider helper is set, update that\ntree row item's value"
        n248 = event-data() -> ("NewVal"=w395:dbl)  [unwired: 1 in]
        n249 = call <vilib>:"NT Write Number.vi"("Numeric"=w395, "Name"=w396) -> ()  [unwired: 9 in, 1 out]
      }
      event "On/Off": Value Change {
        # "When the test mode on/off helper value is set, update that\ntree row item's value"
        n250 = event-data() -> ("NewVal"=w400:bool)  [unwired: 1 in]
        n251 = Boolean To (0,1)(Boolean=w400) -> (0, 1=w399:i16)
        n252 = call <vilib>:"NT Write Number.vi"("Numeric"=w399, "Name"=w398) -> ()  [unwired: 9 in, 1 out]
      }
      event "Rev/Fwd": Value Change {
        # "When the test mode helper value for relays is set, update that\ntree row item's value"
        n253 = event-data() -> ("NewVal.Forward"=w408:bool, "NewVal.Reverse"=w407:bool)  [unwired: 1 in]
        n254 = Boolean To (0,1)(Boolean=w408) -> (0, 1=w404:i16)
        n255 = Boolean To (0,1)(Boolean=w407) -> (0, 1=w406:i16)
        n256 = Negate(x=w406) -> (-x=w405:i16)
        n257 = Add(x=w404, y=w405) -> (x+y=w403:i16)
        n258 = call <vilib>:"NT Write Number.vi"("Numeric"=w403, "Name"=w402) -> ()  [unwired: 9 in, 1 out]
      }
      event "Test Ring": Value Change {
        # "When a test mode helper value is selected from the ring,\nset the tree item's variable to the string value"
        n259 = event-data() -> ("NewVal"=w412:u16)  [unwired: 1 in]
        n260 = property on="Test Ring" class="Ring (strict)"() -> ("Strings []"=w413:string[])  [unwired: 2 in, 2 out]
        n261 = Index Array(array=w413, index=w412) -> (element=w411:string)
        n262 = call <vilib>:"NT Write String.vi"("String"=w411, "Name"=w410) -> ()  [unwired: 9 in, 1 out]
      }
      event "Rec Mode": Value Change {
        # "Update globals for recording mode and path to read log from.\nClear when logging and let NetworkTables set path for vision to\nuse."
        n263 = event-data() -> ("NewVal"=w423:enum32{"Stop", "Record", "Playback"})  [unwired: 1 in]
        n264 = global write "WPI_DashboardLogging Global.vi" "Logging Filename"(path "") -> ()
        n265 = case shown="\"Playback\"" w423 {
          tunnel: w422 -> [_ w425 w433]
          tunnel: [_ _ w432] -> w419
          tunnel: [_ _ w431] -> _
          tunnel: w417 -> [_ _ w429]
          tunnel: cluster{i32, i32} {-250, 170} -> [_ _ w428]
          tunnel: [_ _ T23 {"Image Size"=TRUE, "Image Type"=TRUE, "Pixel Value"=TRUE, "ROI Information"=TRUE, "Zoom Factor"=FALSE} ("Image Information Shown:All Elements")] -> w415
          tunnel: [_ _ TRUE ("Zoom Factor")] -> w414
          frame Default {
          }
          frame "Stop", "Record" {
            # "Place Window too"
            n266 = invoke class="VI" method="FP.Close"(reference=w425) -> (reference out=w424:refnum<vi>)  [unwired: 2 in, 2 out]
            n267 = invoke class="VI" method="Abort VI"(reference=w424) -> ()  [unwired: 2 in, 3 out]
          }
          frame "Playback" {
            n268 = call "Open Playback Panel.vi"("Offset"=w428, "DB VI Ref"=w429, "Playback in"=w433) -> ("Playback out"=w430:refnum<vi>)  [unwired: 8 in]
            n269 = register-events(w430) -> (reference out=w432:refnum<event-registration>, error out=w431:errorcluster)  [unwired: 2 in]
          }
        }
        n270 = global write "WPI_DashboardLogging Global.vi" "Recording"(w423) -> ()
        n271 = property on="Camera Image" class="ImageControl"("Image Information Shown"=w415, "Image Information Visible"=w414) -> ()  [unwired: 2 in, 2 out]
        n272 = call <vilib>:"WPI_DashboardNT Log FieldName Cache.vi"("Operation"=enum16{"Lookup/Add", "Index", "Clear"}."Clear") -> ()  [unwired: 8 in, 3 out]
      }
      event Panel Close {
        w434 = enum32{"Stop", "Record", "Playback"}."Stop" ("Rec Mode")
        # "Playback window has been closed, abort"
        n273 = event-data() -> ()  [unwired: 1 in, 4 out]
        n274 = local write "Rec Mode"(w434) -> ()
        n275 = global write "WPI_DashboardLogging Global.vi" "Recording"(w434) -> ()
      }
      event Panel Close {
        # "Abort playback window and ourself"
        n276 = event-data() -> ()  [unwired: 1 in, 4 out]
        n277 = invoke class="VI" method="FP.Close"(reference=w439) -> (reference out=w438:refnum<vi>)  [unwired: 2 in, 2 out]
        n278 = invoke class="VI" method="Abort VI"(reference=w438) -> (error out=w437:errorcluster)  [unwired: 2 in, 2 out]
        n279 = invoke class="VI" method="Abort VI"(error in=w437) -> ()  [unwired: 2 in, 3 out]
      }
      event "Vision": Value Change {
        # "Enable/Disable Compression slider.\nHW USB is hard-coded into the camera"
        n280 = event-data() -> ("NewVal"=w445:u16)  [unwired: 1 in]
        n281 = Equal?(x=w445, y=u32 2 ("milliseconds to wait")) -> (x = y?=w443:bool)
        n282 = Select(t=T24."Disabled and Grayed Out" ("Disabled"), s=w443, f=T24."Enabled" ("Disabled")) -> (s? t:f=w440:T24)
        n283 = property on="Compression" class="Slide (strict)"("DisabledEnum"=w440) -> ()  [unwired: 2 in, 2 out]
      }
    }
  }
  n284 = while {
    tunnel: w40 -> [w448]
    i -> [w451]
    stop <- FALSE stop-if-true
    n285 = Wait (ms)(milliseconds to wait=u32 100) -> ()  [unwired: 1 out]
    n286 = case shown="\"Playback\"" "Rec Mode" {
      tunnel: w451 -> [_ _ w466]
      tunnel: [u32 2829099 ("Base Color") u32 11141120 ("Target Color") w455] -> w447
      frame "Stop", Default {
        # "Reset the color, extra updates don't cost much"
      }
      frame "Record" {
      }
      frame "Playback" {
        # "Playback"
        n287 = Quotient & Remainder(x=w466, y=u32 50 ("milliseconds to wait")) -> (x-y*floor(x/y)=w462:u32)  [unwired: 1 out]
        n288 = Divide(x=w462, y=u32 50 ("milliseconds to wait")) -> (x/y=w459:dbl)
        n289 = Multiply(x=6.283185307179586, y=w459) -> (x*y=w464:dbl)
        n290 = Sine(x=w464) -> (sin(x)=w463:dbl)
        n291 = Absolute Value(x=w463) -> (abs(x)=w456:dbl)
        n292 = call "Interpolate RGB Color.vi"("Proportion"=w456, "Target Color"=u32 30976, "Base Color"=u32 2829099) -> ("Result Color"=w455:u32)  [unwired: 8 in]
      }
    }
    n293 = property class="Pane"(reference=w448, "PaneColor"=w447) -> ()  [unwired: 1 in, 2 out]
  }
  n294 = TCP Create Listener(10:u16 1741 ("timeout ms (25000)")) -> (3:w3:refnum<k5>)  [unwired: 4 in, 2 out]
  n295 = while {
    tunnel: w3 -> [w468]
    stop <- FALSE stop-if-true
    n296 = TCP Wait On Listener(11:w468) -> (4:w467:refnum<k5>)  [unwired: 3 in, 4 out]
    n297 = local write "TCP"(w467) -> ()
  }
  n298 = property on="On/Off" class="Bool (strict)"("Visible"=w8) -> ()  [unwired: 2 in, 2 out]
  n299 = property on="Motor" class="Clust (strict)"("Visible"=w8) -> ()  [unwired: 2 in, 2 out]
  n300 = property on="Progress" class="Clust (strict)"("Visible"=w8) -> ()  [unwired: 2 in, 2 out]
  n301 = property on="Test Ring" class="Ring (strict)"("Visible"=w8) -> ()  [unwired: 2 in, 2 out]
  n302 = property on="Rev/Fwd" class="Clust (strict)"("Visible"=w8) -> ()  [unwired: 2 in, 2 out]
  n303 = property on="Camera Settings" class="Clust (strict)"("Visible"=w8) -> ()  [unwired: 2 in, 2 out]
  n304 = local write "DB Camera Config"(w8) -> ()
  n305 = global write "WPI_DashboardLogging Global.vi" "Recording"(w34) -> ()
  n306 = local write "Rec Mode"(w34) -> ()
